vi "Main.vi"(8 "error in (no error)":errorcluster, 11 "Module_Refs":T2={"ModuleName"=enum."Controller", "Queue"=refnum, "user event"=refnum, "VI Refnum"=refnum, "ShowFP"=FALSE, "StatesTracking Enabled"=FALSE}) -> (0 "error out":errorcluster)   [LabVIEW 2021, in "Sound Manager.lvlib"]
uses:
  Sound Manager.lvlib
  Architecture/Typedefs/Module References.ctl
  Architecture/Typedefs/Enum_Module_Name.ctl
  Architecture/Typedefs/Message.ctl
  Typedefs/Sound Effects.ctl
  Typedefs/States.ctl
  Typedefs/Sound Data.ctl
  <vilib>/sound2/lvsound2.llb/Sound Output Task ID.ctl
  Typedefs/Config.ctl
  <vilib>/event_ctls.llb/usereventprio.ctl
  Architecture/Modules/Configuration/Typedefs/App Cfg DVR.ctl
  Architecture/Typedefs/Application Configuration.ctl
  Architecture/Modules/Module Template/Typedefs/Config.ctl
  Architecture/Modules/Core UI/Typedefs/Config.ctl
  Utilities/Globales Snake.vi
  SubVIs/Read Sound ConfigurationI.vi
  Architecture/Architecture.lvlib
  Architecture/Modules/Configuration/Configuration.lvlib
  Architecture/Modules/Module Template/Module Template.lvlib
  Architecture/Modules/Core UI/Board Game.lvlib
panel:
  out "BackGround Track":string
  in  "Next":bool
  in  "Multicolumn Listbox":i32(listbox)
  in  "Stop Sound Effect":bool
  in  "Play Sound Effect":bool
  in  "Sound Effect":T1
  in  "Background music":bool
  in  "Load Config":bool
  out "Message":string
  in  "Stop App":bool
  in  "Stop Module":bool
  # "#Architecture\n\nPlace inside this box all visible data."
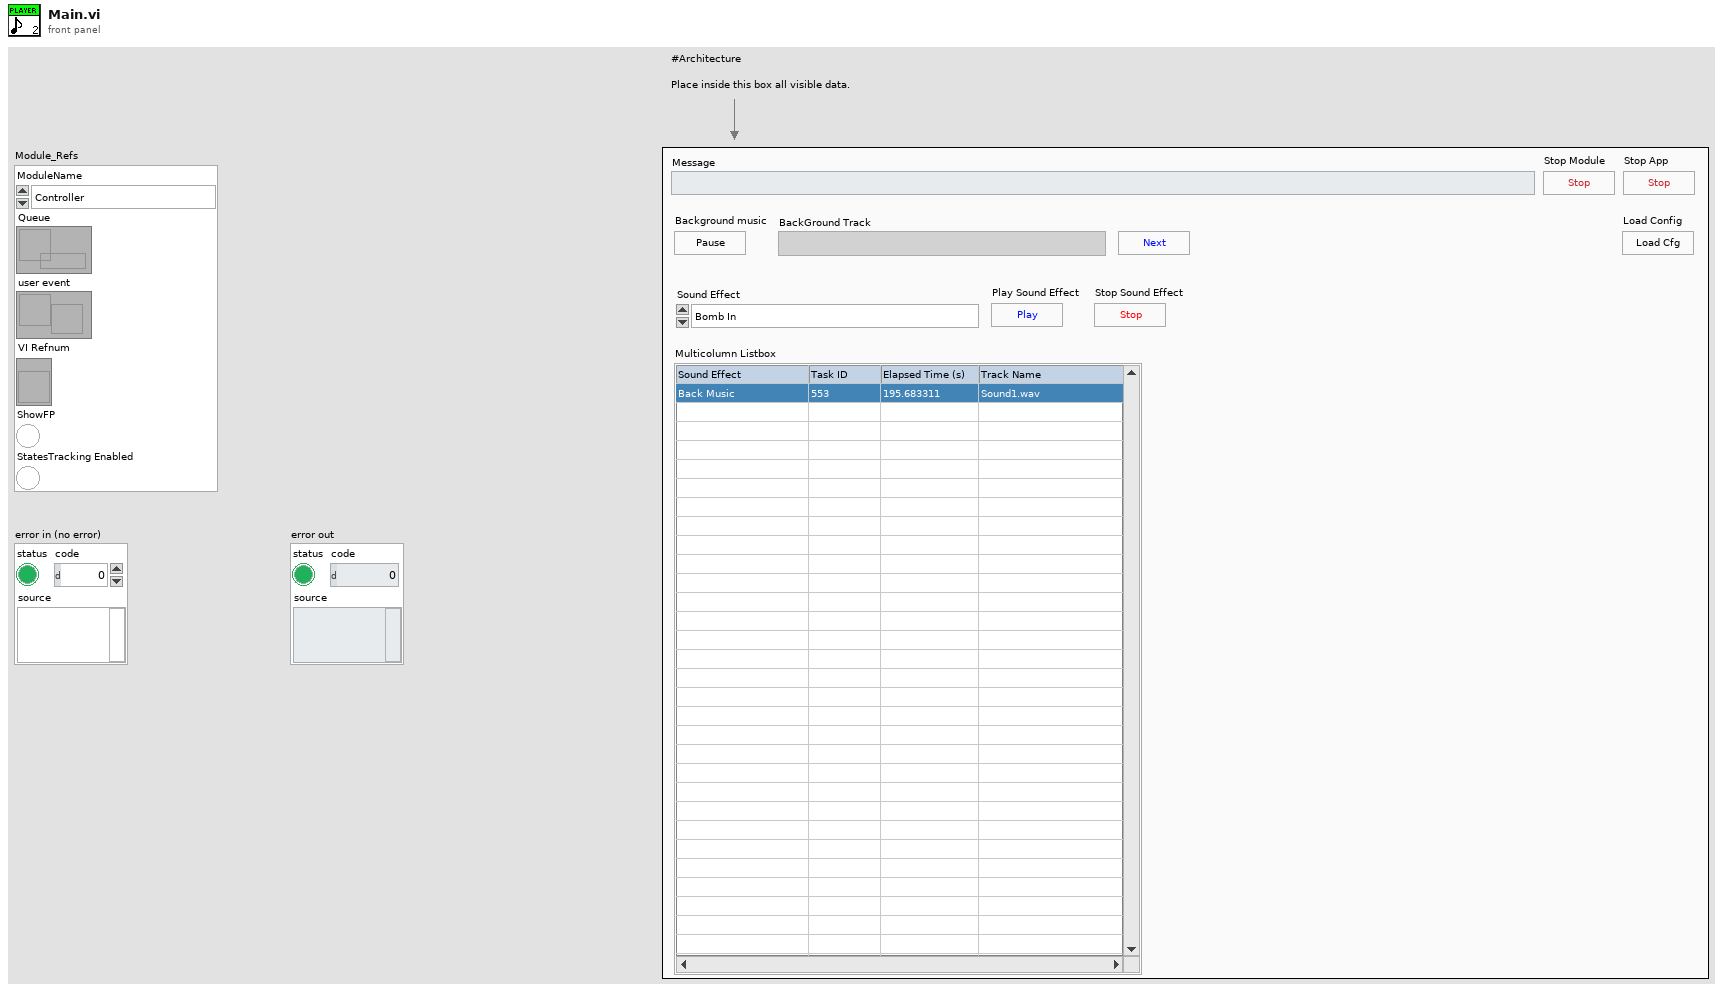
[diagram p1: front panel]
types:
  T1 = typedef "Sound Manager.lvlib/Sound Effects.ctl" = enum16{"Bomb In", "Bomb Out", "Bomb Touched", "Game Over", "Victory", "Eat", "10 Fruits", "Eat2", "Eat3", "Eat4", "MaxShield", "Shield", "10p", "Grape In", "Grape Out", "20p", "30p", "40p", "50p", "60p", "70p", "80p", "90p", "100p", "All shields cracked", "Mouse In", "Mouse Out", "Mouse Eaten", "Grape Eaten", "States Recover", "Broken Shield", "Bonus", "Happy Time", "explode", "Game over musica", "Back Music", "Shield Catch", "Evil lough", "Cricket In", "Cricket eaten", "Lets Go", "Jump1", "Jump2", "Jump3", "Unstoppable", "Troll Music", "winner", "menu"}
  T2 = typedef "Architecture.lvlib/Module References.ctl" = cluster{"ModuleName":T3, "Queue":refnum<queue>, "user event":refnum<user-event>, "VI Refnum":refnum<vi>, "ShowFP":bool, "StatesTracking Enabled":bool}
  T3 = typedef "Configuration.lvlib/Enum_Module_Name.ctl" = enum16{"Configuration", "Error_Handler", "Log", "Database", "Controller", "UI Module", "Sound Manager"}
  T4 = typedef "Sound Manager.lvlib/States.ctl" = cluster{"Module_Refs":T2, "Response Data":variant, "Music Paused":bool, "Tasks":T5[], "Config":T7, "Background Track":string}
  T5 = typedef "Sound Manager.lvlib/Sound Data.ctl" = cluster{"Sound Effect":T1, "Task ID":T6, "Init":timestamp, "Track Name":string}
  T6 = typedef "Sound Output Task ID.ctl" = u32
  T7 = typedef "Sound Manager.lvlib/Config.ctl" = cluster{"Sound Library Path":path, "dyn sounds path":path}
  T8 = enum32{"Invalid", "Standard", "Closed", "Hidden", "Minimized", "Maximized"}
  T9 = typedef "Error_Manager.lvlib/LogRotate.lvclass/LogData.ctl" = cluster{"error in":errorcluster, "replacements":string[], "Time Stamp":timestamp}
  T10 = typedef "Configuration.lvlib/App Cfg DVR.ctl" = refnum<data-value>
  T11 = typedef "usereventprio.ctl" = enum32{"high priority", "normal priority"}
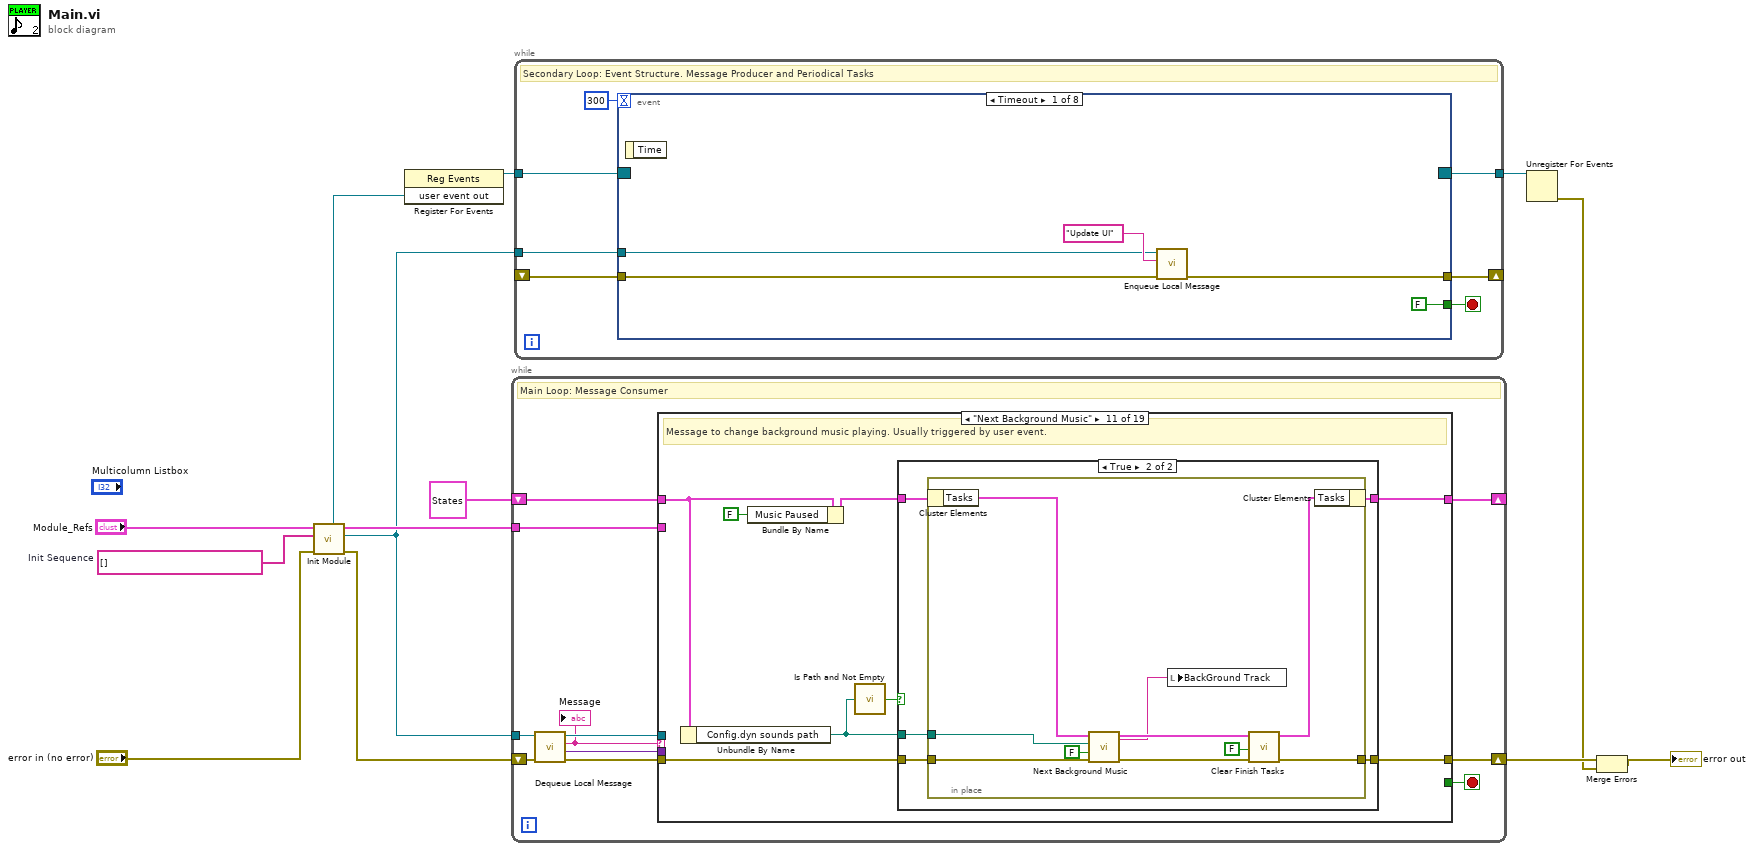
[diagram p0: block diagram]
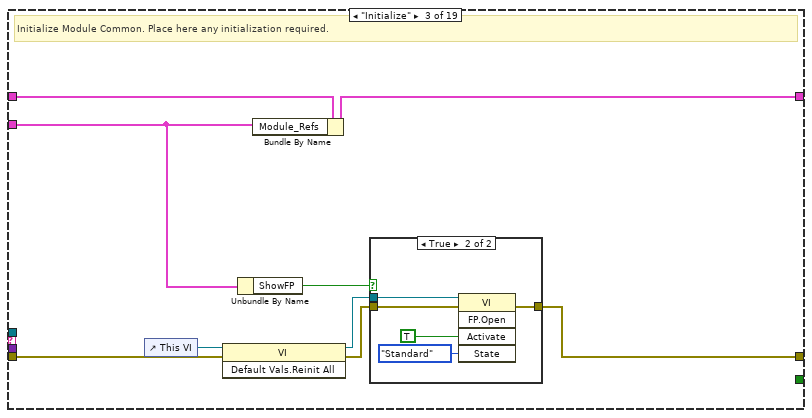
[diagram p4: hidden frame]
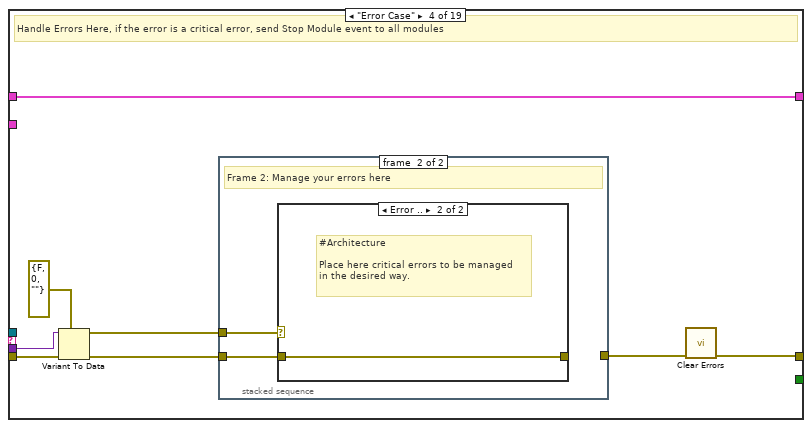
[diagram p6: hidden frame]
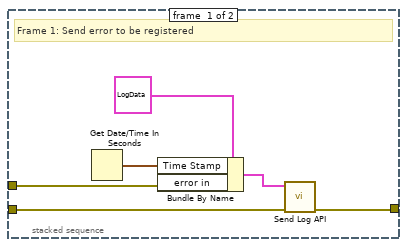
[diagram p7: hidden frame]
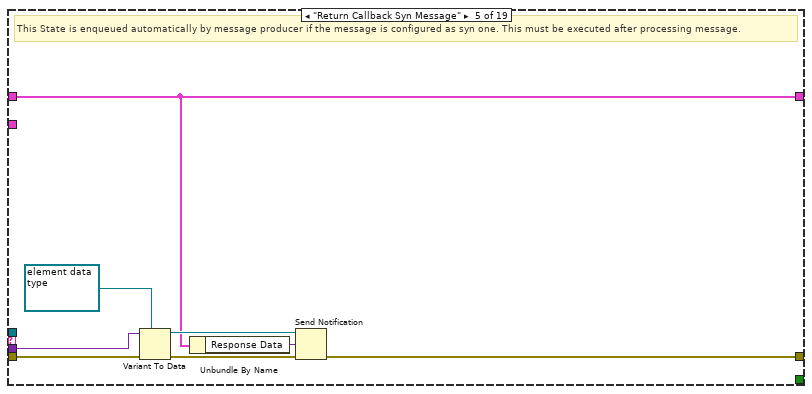
[diagram p9: hidden frame]
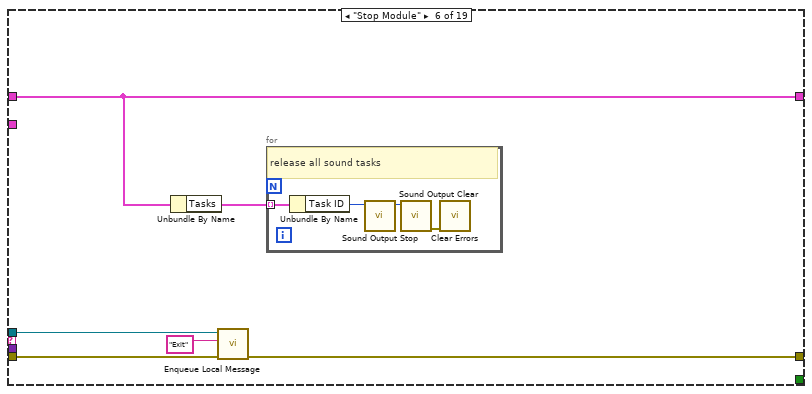
[diagram p10: hidden frame]
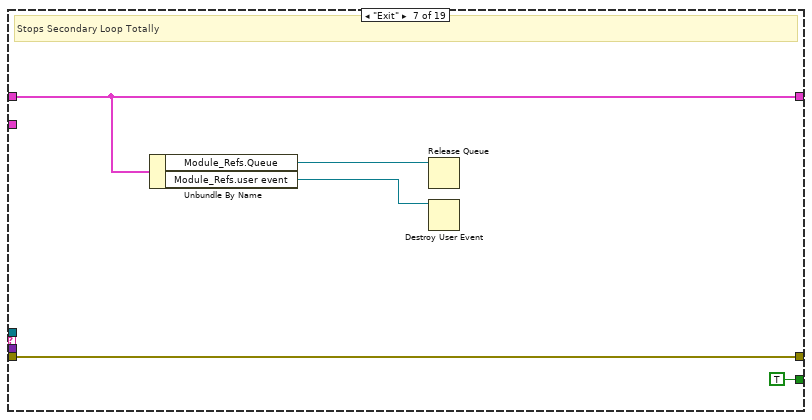
[diagram p11: hidden frame]
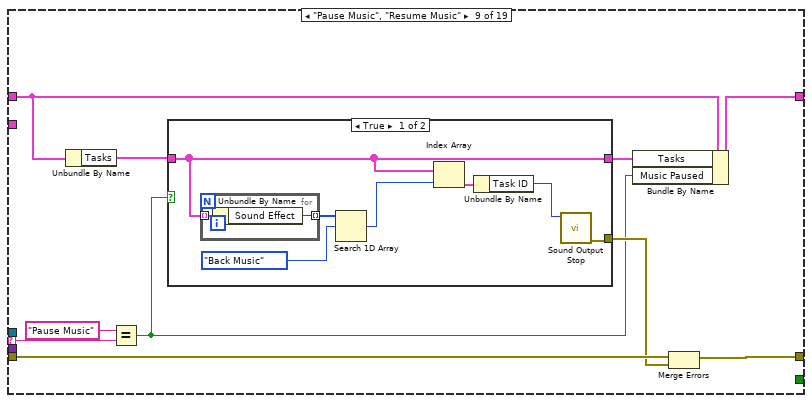
[diagram p13: hidden frame]
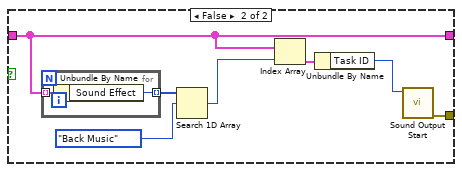
[diagram p14: hidden frame]
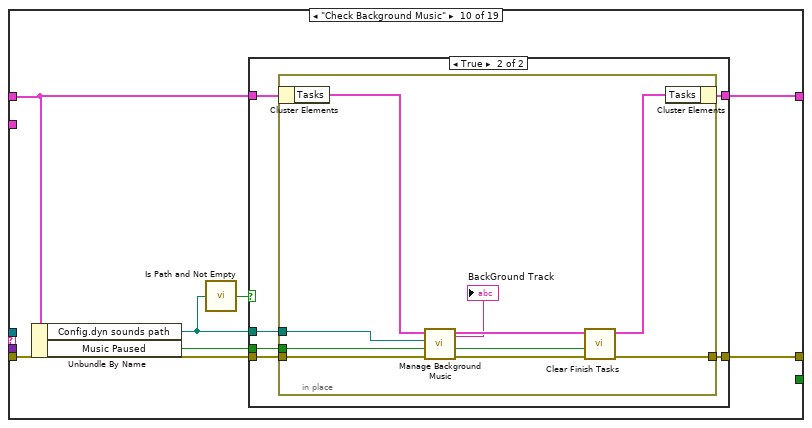
[diagram p15: hidden frame]
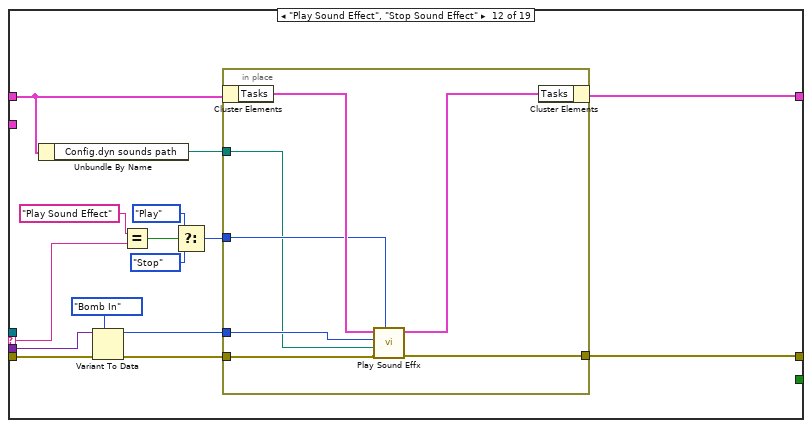
[diagram p18: hidden frame]
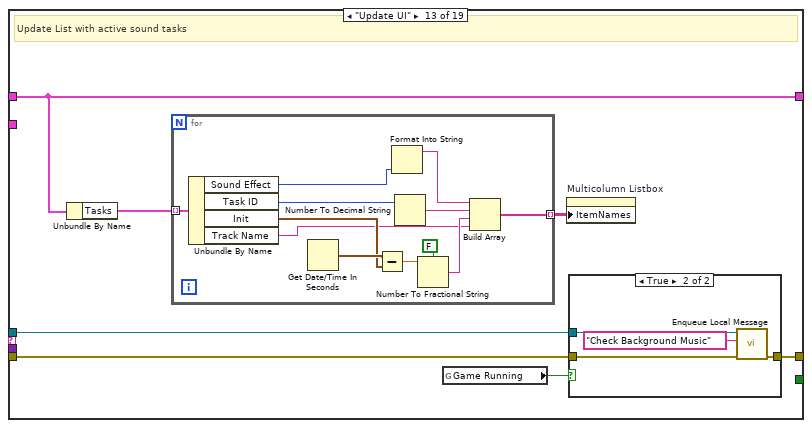
[diagram p19: hidden frame]
diagram:
  w11 = string[] []  # Init Sequence
  n1 = call "Init Module.vi"("error in (no error)"="error in (no error)", "Init Sequence"=w11, "Module Refs"="Module_Refs") -> ("error out"=w13:errorcluster, "queue out"=w2:refnum<queue>, "Module Refs Out"=w4:T2, "user event out"=w3:refnum<user-event>)  [unwired: 5 in]
  n2 = register-events(w3) -> (reference out=w10:refnum<event-registration>)  [unwired: 2 in, 1 out]
  n3 = while {
    shift-right: [w23] -> _
    shift-left: T4 {"Module_Refs"={"ModuleName"=enum."Controller", "Queue"=refnum, "user event"=refnum, "VI Refnum"=refnum, "ShowFP"=FALSE, "StatesTracking Enabled"=FALSE}, "Response Data"=variant, "Music Paused"=FALSE, "Tasks"=[], "Config"={"Sound Library Path"=path "", "dyn sounds path"=path ""}, "Background Track"=""} ("SM Data") -> [w24]
    shift-right: [w22] -> w8
    shift-left: w13 -> [w20]
    tunnel: w2 -> [w21]
    tunnel: w4 -> [w14]
    stop <- w15 stop-if-true
    # "Main Loop: Message Consumer"
    n4 = call "Dequeue Local Message.vi"("error in"=w20, "Msg queue in"=w21) -> ("error out"=w19:errorcluster, "Data"=w16:variant, "Message"=w17:string, "queue out"=w18:refnum<queue>)  [unwired: 6 in]
    "Message" <- w17
    n5 = case shown="\"Next Background Music\"" w17 {
      selector: w17 -> [_ _ _ _ _ _ _ _ w94 _ _ w171 _ _ w212 _ _ _ w256]
      tunnel: w24 -> [w26 w28 w37 w51 w63 w71 w82 w86 w92 w118 w144 w175 w192 w211 w219 w224 w229 w247 w261]
      tunnel: [w26 w28 w35 w51 w63 w71 w82 w86 w95 w117 w143 w173 w192 w211 w219 w224 w225 w247 w261] -> w23
      tunnel: w19 -> [w25 w27 w36 w50 w69 w75 w84 w85 w96 w120 w146 w178 w188 w210 w216 w223 w228 w246 w260]
      tunnel: [w25 w27 w31 w44 w68 w74 w84 w85 w89 w119 w145 w172 w187 w210 w213 w222 w226 w246 w250] -> w22
      tunnel: w18 -> [_ _ _ _ _ w73 _ _ _ _ _ _ w189 _ w214 w221 _ _ w257]
      tunnel: w16 -> [_ _ _ w49 w66 _ _ _ _ _ _ w177 _ _ w215 _ w227 _ w258]
      tunnel: [_ _ _ _ _ _ TRUE _ _ _ _ _ _ _ _ _ _ _ _] -> w15
      tunnel: w14 -> [_ _ w34 _ _ _ _ _ _ _ _ _ _ _ _ _ _ _ _]
      frame "--------State Machine Arquitechture Operations--------" {
      }
      frame "Idle", Default {
        # "Use this state to make iterations if required."
      }
      frame "Initialize" {
        # "Initialize Module Common. Place here any initialization required."
        n6 = control-ref of="This VI"() -> (w29:refnum<vi>)
        n7 = invoke class="VI" method="Default Vals.Reinit All"(reference=w29, error in=w36) -> (reference out=w32:refnum<vi>, error out=w33:errorcluster)  [unwired: 1 in, 1 out]
        n8 = Unbundle By Name(w34) -> ("ShowFP"=w30:bool)
        n9 = Bundle By Name(cluster=w37, "Module_Refs"=w34) -> (w35:T4)
        n10 = case shown="True" w30 {
          tunnel: w33 -> [w38 w43]
          tunnel: [w38 w42] -> w31
          tunnel: w32 -> [_ w41]
          frame False {
          }
          frame True {
            n11 = invoke class="VI" method="FP.Open"(reference=w41, error in=w43, "Activate"=TRUE ("Activate?"), "State"=T8."Standard") -> (error out=w42:errorcluster)  [unwired: 1 in, 4 out]
          }
        }
      }
      frame "Error Case" {
        # "Handle Errors Here, if the error is a critical error, send Stop Module event to all modules"
        n12 = Variant To Data(error in=w50, type=errorcluster {"status"=FALSE, "code"=0, "source"=""} ("error constant"), Variant=w49) -> (data=w45:errorcluster, error out=w47:errorcluster)
        n13 = stacked-sequence {
          tunnel: w47 -> [w57 w59]
          tunnel: [w56 _] -> w46
          tunnel: w45 -> [w54 w58]
          frame #0 {
            # "Frame 1: Send error to be registered"
            n14 = Get Date/Time In Seconds() -> (seconds since 1Jan1904=w53:timestamp)
            n15 = Bundle By Name(cluster=T9 {"error in"={"status"=FALSE, "code"=0, "source"=""}, "replacements"=[], "Time Stamp"=timestamp(0 s since 1904-01-01)} ("Data"), "Time Stamp"=w53, "error in"=w54) -> (w52:T9)
            n16 = call "Send Log API.vi"("error in (no error)"=w57, "Data"=w52) -> ("error out"=w56:errorcluster)  [unwired: 9 in]
          }
          frame #1 {
            # "Frame 2: Manage your errors here"
            n17 = case shown="Error .." w58 {
              tunnel: [w60 w61] -> _
              tunnel: w59 -> [w60 w61]
              frame No Error {
              }
              frame Error {
                # "#Architecture \n\nPlace here critical errors to be managed \nin the desired way."
              }
            }
          }
        }
        n18 = call <vilib>:"Clear Errors.vi"("error in (no error)"=w46) -> ("error out"=w44:errorcluster)  [unwired: 5 in, 1 out]
      }
      frame "Return Callback Syn Message" {
        # "This State is enqueued automatically by message producer if the message is configured as syn one. This must be executed after processing message."
        n19 = Variant To Data(error in=w69, type=refnum<notifier> refnum ("notifier out"), Variant=w66) -> (data=w64:refnum<notifier>, error out=w67:errorcluster)
        n20 = Unbundle By Name(w63) -> ("Response Data"=w62:variant)
        n21 = Send Notification(notification=w62, notifier=w64, error in (no error)=w67) -> (error out=w68:errorcluster)  [unwired: 1 out]
      }
      frame "Stop Module" {
        n22 = Unbundle By Name(w71) -> ("Tasks"=w70:T5[])
        n23 = call "Enqueue Local Message.vi"("error in"=w75, "Message"="Exit", "Msg queue in"=w73) -> ("error out"=w74:errorcluster)  [unwired: 7 in, 1 out]
        n24 = for {
          tunnel: w70 -> [w77] mode=indexing
          # "release all sound tasks"
          n25 = Unbundle By Name(w77) -> ("Task ID"=w76:T6)
          n26 = call <vilib>:"Sound Output Stop.vi"("task ID"=w76) -> ("task ID out"=w78:T6)  [unwired: 9 in, 1 out]
          n27 = call <vilib>:"Sound Output Clear.vi"("task ID"=w78) -> ("error out"=w79:errorcluster)  [unwired: 10 in]
          n28 = call <vilib>:"Clear Errors.vi"("error in (no error)"=w79) -> ()  [unwired: 5 in, 2 out]
        }
      }
      frame "Exit" {
        # "Stops Secondary Loop Totally"
        n29 = Unbundle By Name(w82) -> ("Module_Refs.Queue"=w81:refnum<queue>, "Module_Refs.user event"=w80:refnum<user-event>)
        n30 = Release Queue(queue=w81) -> ()  [unwired: 2 in, 3 out]
        n31 = Destroy User Event(user event=w80) -> ()  [unwired: 1 in, 1 out]
      }
      frame "--------------State Machine Custom States-------------" {
      }
      frame "Pause Music", "Resume Music" {
        n32 = Unbundle By Name(w92) -> ("Tasks"=w91:T5[])
        n33 = Equal?(x="Pause Music", y=w94) -> (x = y?=w87:bool)
        n34 = case shown="True" w87 {
          tunnel: w91 -> [w99 w109]
          tunnel: [w99 w109] -> w90
          tunnel: [w97 w107] -> w88
          frame True {
            n35 = for {
              tunnel: w99 -> [w105] mode=indexing
              tunnel: [w104] -> w101 mode=indexing
              n36 = Unbundle By Name(w105) -> ("Sound Effect"=w104:T1)
            }
            n37 = Search 1D Array(1D array=w101, element=Sound_Effects."Back Music") -> (index of element=w100:i32)  [unwired: 1 in]
            n38 = Index Array(array=w99, index=w100) -> (element=w103:T5)
            n39 = Unbundle By Name(w103) -> ("Task ID"=w98:T6)
            n40 = call <vilib>:"Sound Output Stop.vi"("task ID"=w98) -> ("error out"=w97:errorcluster)  [unwired: 9 in, 1 out]
          }
          frame False {
            n41 = for {
              tunnel: w109 -> [w114] mode=indexing
              tunnel: [w113] -> w111 mode=indexing
              n42 = Unbundle By Name(w114) -> ("Sound Effect"=w113:T1)
            }
            n43 = Search 1D Array(1D array=w111, element=Sound_Effects."Back Music" ("Sound Effect")) -> (index of element=w110:i32)  [unwired: 1 in]
            n44 = Index Array(array=w109, index=w110) -> (element=w112:T5)
            n45 = Unbundle By Name(w112) -> ("Task ID"=w108:T6)
            n46 = call <vilib>:"Sound Output Start.vi"("task ID"=w108) -> ("error out"=w107:errorcluster)  [unwired: 9 in, 1 out]
          }
        }
        n47 = Bundle By Name(cluster=w92, "Tasks"=w90, "Music Paused"=w87) -> (w95:T4)
        n48 = Merge Errors(w96, w88) -> (w89:errorcluster)
      }
      frame "Check Background Music" {
        n49 = Unbundle By Name(w118) -> ("Config.dyn sounds path"=w116:path, "Music Paused"=w121:bool)
        n50 = call <vilib>:"Is Path and Not Empty.vi"("path"=w116) -> ("Is Path and Not Empty?"=w115:bool)  [unwired: 4 in]
        n51 = case shown="True" w115 {
          tunnel: w121 -> [_ w129]
          tunnel: w120 -> [w122 w128]
          tunnel: [w122 w124] -> w119
          tunnel: w118 -> [w123 w127]
          tunnel: [w123 w126] -> w117
          tunnel: w116 -> [_ w125]
          frame False {
          }
          frame True {
            n52 = in-place {
              in-place-border: w129 -> [w131]
              in-place-border: w128 -> [w136]
              in-place-border: w125 -> [w135]
              in-place-border: [w138] -> w124
              n53 = in-place-cluster #1(w127) -> ("Tasks"=w134:T5[])
              n54 = call "Manage Background Music.vi"("error in (no error)"=w136, "Music Paused"=w131, "Dyn Sounds Path"=w135, "Sounds"=w134) -> ("error out"=w137:errorcluster, "Sounds Out"=w133:T5[], "BackGround Track"=→"BackGround Track":string)  [unwired: 5 in]
              n55 = call "Clear Finish Tasks.vi"("error out"=w137, "Music Paused"=w131, "Sounds In"=w133) -> ("error out"=w138:errorcluster, "Sounds Out"=w132:T5[])  [unwired: 7 in]
              n56 = in-place-cluster #1("Tasks"=w132) -> (w126:T4)
            }
          }
        }
      }
      frame "Next Background Music" {
        # "Message to change background music playing. Usually triggered by user event."
        n57 = Unbundle By Name(w144) -> ("Config.dyn sounds path"=w142:path)
        n58 = Bundle By Name(cluster=w144, "Music Paused"=FALSE) -> (w140:T4)
        n59 = call <vilib>:"Is Path and Not Empty.vi"("path"=w142) -> ("Is Path and Not Empty?"=w141:bool)  [unwired: 4 in]
        n60 = case shown="True" w141 {
          tunnel: w146 -> [w147 w153]
          tunnel: [w147 w152] -> w145
          tunnel: w140 -> [w148 w151]
          tunnel: [w148 w150] -> w143
          tunnel: w142 -> [_ w149]
          frame False {
          }
          frame True {
            n61 = in-place {
              in-place-border: w153 -> [w156]
              in-place-border: [w161] -> w152
              in-place-border: w149 -> [w157]
              n62 = in-place-cluster #2(w151) -> ("Tasks"=w159:T5[])
              n63 = call "Next Background Music.vi"("error in (no error)"=w156, "Music Paused"=FALSE, "Dyn Sounds Path"=w157, "Sounds"=w159) -> ("error out"=w163:errorcluster, "Sounds Out"=w162:T5[], "BackGround Track"=w158:string)  [unwired: 5 in]
              n64 = local write "BackGround Track"(w158) -> ()
              n65 = call "Clear Finish Tasks.vi"("error out"=w163, "Music Paused"=FALSE, "Sounds In"=w162) -> ("error out"=w161:errorcluster, "Sounds Out"=w160:T5[])  [unwired: 7 in]
              n66 = in-place-cluster #2("Tasks"=w160) -> (w150:T4)
            }
          }
        }
      }
      frame "Play Sound Effect", "Stop Sound Effect" {
        n67 = Unbundle By Name(w175) -> ("Config.dyn sounds path"=w174:path)
        n68 = Variant To Data(error in=w178, type=Sound_Effects."Bomb In" ("Sound Effect Off"), Variant=w177) -> (data=w164:T1, error out=w176:errorcluster)
        n69 = Equal?(x="Play Sound Effect", y=w171) -> (x = y?=w169:bool)
        n70 = Select(t=enum16{"Play", "Stop"}."Play" ("event"), s=w169, f=enum16{"Play", "Stop"}."Stop" ("event")) -> (s? t:f=w166:enum16{"Play", "Stop"})
        n71 = in-place {
          in-place-border: w176 -> [w185]
          in-place-border: w174 -> [w180]
          in-place-border: [w179] -> w172
          in-place-border: w166 -> [w182]
          in-place-border: w164 -> [w181]
          n72 = in-place-cluster #3(w175) -> ("Tasks"=w184:T5[])
          n73 = call "Play Sound Effx.vi"("event"=w182, "error in (no error)"=w185, "path"=w180, "Sound Effect Off"=w181, "Sounds In"=w184) -> ("error out"=w179:errorcluster, "Sounds Out"=w183:T5[])  [unwired: 5 in]
          n74 = in-place-cluster #3("Tasks"=w183) -> (w173:T4)
        }
      }
      frame "Update UI" {
        # "Update List with active sound tasks"
        n75 = Unbundle By Name(w192) -> ("Tasks"=w191:T5[])
        n76 = for {
          tunnel: w191 -> [w209] mode=indexing
          tunnel: [w199] -> w190 mode=indexing
          n77 = Unbundle By Name(w209) -> ("Sound Effect"=w208:T1, "Task ID"=w206:T6, "Init"=w203:timestamp, "Track Name"=w198:string)
          n78 = Get Date/Time In Seconds() -> (seconds since 1Jan1904=w204:timestamp)
          n79 = Subtract(x=w204, y=w203) -> (x-y=w202:dbl)
          n80 = Format Into String(w208) -> (resulting string=w207:string)  [unwired: 3 in, 1 out]
          n81 = Number To Decimal String(number=w206) -> (decimal integer string=w205:string)  [unwired: 1 in]
          n82 = Number To Fractional String(use system decimal point (T)=FALSE, number=w202) -> (F-format string=w200:string)  [unwired: 2 in]
          n83 = Build Array(w207, w205, w200, w198) -> (w199:string[])
        }
        n84 = global read "Globales Snake.vi" "Game Running"() -> (w186:bool)
        n85 = property on="Multicolumn Listbox" class="MCListbox (strict)"("ItemNames"=w190) -> ()  [unwired: 2 in, 2 out]
        n86 = case shown="True" w186 {
          tunnel: w189 -> [_ w196]
          tunnel: w188 -> [w193 w195]
          tunnel: [w193 w194] -> w187
          frame False {
          }
          frame True {
            n87 = call "Enqueue Local Message.vi"("error in"=w195, "Message"="Check Background Music", "Msg queue in"=w196) -> ("error out"=w194:errorcluster)  [unwired: 7 in, 1 out]
          }
        }
      }
      frame "--------------Dynamic Events Messages----------------" {
      }
      frame "Message: Check Background Music", "Message: MyMessage", "Message: Next Background Music", "Message: Pause Music", "Message: Play Sound Effect", "Message: Resume Music", "Message: Stop Sound Effect" {
        n88 = Match Pattern(string=w212, regular expression="Message: ") -> (after substring=w217:string)  [unwired: 1 in, 3 out]
        n89 = call "Enqueue Local Message.vi"("error in"=w216, "Data"=w215, "Message"=w217, "Msg queue in"=w214) -> ("error out"=w213:errorcluster)  [unwired: 6 in, 1 out]
      }
      frame "Message: Stop Module" {
        n90 = call "Enqueue Local Message.vi"("error in"=w223, "Message"="Stop Module", "Msg queue in"=w221) -> ("error out"=w222:errorcluster)  [unwired: 7 in, 1 out]
      }
      frame "Message: Load Config" {
        # "Message used to receive configuration from a configuration module. Decode dedicated typedef and save it into SM Data"
        n91 = disable-structure shown="Simulation==False, Default" {
          disable-tunnel: w229 -> [w238 w244]
          disable-tunnel: w228 -> [w237 w245]
          disable-tunnel: w227 -> [w236 _]
          disable-tunnel: [w230 _] -> w226
          disable-tunnel: [_ w245] -> _
          disable-tunnel: [w234 w243] -> w225
          frame condition #0 (active) {
            n92 = Variant To Data(error in=w237, type=T10 refnum ("App Cfg DVR"), Variant=w236) -> (data=w233:T10, error out=w232:errorcluster)
            n93 = call-poly "POLY Read Configuration API.vi"("error constant"=w232, "App Cfg DVR"=w233) -> ("error out"=w230:errorcluster, "Sound Manager Config"=w231:T7)  [unwired: 8 in]
            n94 = Bundle By Name(cluster=w238, "Config"=w231) -> (w234:T4)
          }
          frame condition #1 {
            n95 = call <vilib>:"Application Directory.vi"() -> ("Application Directory"=w242:path)
            n96 = Build Path(base path=w242, name or relative path=path "Resources/sounds/%s.wav") -> (appended path=w240:path)
            n97 = Strip Path(path=w240) -> (stripped path=w239:path)  [unwired: 1 out]
            n98 = Bundle By Name(cluster=w244, "Config.Sound Library Path"=w239, "Config.dyn sounds path"=w240) -> (w243:T4)
          }
        }
      }
      frame "------------Synchronous Event Messages--------------" {
      }
      frame "SynMessage: MySynMessage" {
        # "Use this case as a handler for Synchronous messages. This state queues a message for the desired"
        n99 = call "Extract Synchronous Data.vi"("error in 2"=w260, "Variant"=w258) -> ("error in"=w259:errorcluster, "Data Out"=w253:variant, "notifier out"=w248:refnum<notifier>)  [unwired: 7 in]
        n100 = Match Pattern(string=w256, regular expression="SynMessage: ") -> (after substring=w254:string)  [unwired: 1 in, 3 out]
        n101 = call "Enqueue Local Message.vi"("error in"=w259, "Data"=w253, "Message"=w254, "Msg queue in"=w257) -> ("error out"=w252:errorcluster, "queue out"=w251:refnum<queue>)  [unwired: 6 in]
        n102 = call "Enqueue Local Message.vi"("error in"=w252, "Data"=w248, "Message"="Return Callback Syn Message", "Msg queue in"=w251) -> ("error out"=w250:errorcluster)  [unwired: 6 in, 1 out]
      }
    }
  }
  n103 = while {
    tunnel: w10 -> [w268]
    tunnel: w2 -> [w265]
    tunnel: [w264] -> w9
    shift-right: [w262] -> _
    shift-left: _ -> [w263]
    stop <- w266 stop-if-true
    # "Secondary Loop: Event Structure. Message Producer and Periodical Tasks"
    n104 = event shown="[0] Timeout" {
      selector: w268 -> [_ _ _ _ _ _ _ _]
      dyn-events: [_ _ _ _ _ _ _ _] -> w264
      timeout: 300 -> [_ _ _ _ _ _ _ _]
      tunnel: [FALSE w280 TRUE _ _ _ _ _] -> w266
      tunnel: w265 -> [w269 w285 w287 _ _ _ _ _]
      tunnel: w263 -> [w270 w284 w290 w292 w301 w309 w317 w324]
      tunnel: [w271 w283 w288 w291 w300 w308 w318 w323] -> w262
      event Timeout {
        n105 = event-data() -> ()  [unwired: 1 in, 1 out]
        n106 = call "Enqueue Local Message.vi"("error in"=w270, "Message"="Update UI", "Msg queue in"=w269) -> ("error out"=w271:errorcluster)  [unwired: 7 in, 1 out]
      }
      event User Event {
        # "Send message to local queue. \n(Message Consumer)"
        # "Processes an external event and enqueues a message to the local queue. It can be synchronous (with response) or NOT."
        n107 = event-data() -> ("syn"=w277:bool, "Message"=w279:string, "Data"=w282:variant)  [unwired: 1 in]
        n108 = Select(t="SynMessage: " ("string"), s=w277, f="Message: " ("string")) -> (s? t:f=w274:string)
        n109 = Concatenate Strings(w274, w279) -> (w281:string)
        n110 = call "Enqueue Local Message.vi"("error in"=w284, "Data"=w282, "Message"=w281, "Msg queue in"=w285) -> ("error out"=w283:errorcluster)  [unwired: 6 in, 1 out]
        n111 = Equal?(x=w279, y="Stop Module") -> (x = y?=w280:bool)
      }
      event "Stop Module": Value Change {
        n112 = event-data() -> ()  [unwired: 1 in, 1 out]
        n113 = call "Enqueue Local Message.vi"("error in"=w290, "Message"="Stop Module", "Msg queue in"=w287) -> ("error out"=w288:errorcluster)  [unwired: 7 in, 1 out]
      }
      event "Stop App": Value Change {
        w294 = TRUE  # All Modules
        # "Send Stop To All Modules"
        n114 = event-data() -> ()  [unwired: 1 in, 1 out]
        n115 = call "Send Message Modules.vi"("All Modules"=w294, "Error In"=w292, "Message"="Stop Module") -> ("error in (no error)"=w291:errorcluster)  [unwired: 8 in]
      }
      event "Load Config": Value Change {
        n116 = event-data() -> ()  [unwired: 1 in, 1 out]
        n117 = To Variant(anything=T10 refnum ("App Cfg DVR")) -> (Variant=w298:variant)
        n118 = call "Send Message Module.vi"("priority (normal)"=usereventprio."high priority", "Error In"=w301, "Data"=w298, "Message"="Load Config", "Target ModuleName In"=Enum_Module_Name."Sound Manager" ("ModuleName")) -> ("error in (no error)"=w300:errorcluster)  [unwired: 6 in]
      }
      event "Background music": Value Change {
        n119 = event-data() -> ("NewVal"=w306:bool)  [unwired: 1 in]
        n120 = Select(t="Pause Music", s=w306, f="Resume Music") -> (s? t:f=w303:string)
        n121 = call "Send Message Module.vi"("priority (normal)"=usereventprio."normal priority", "Error In"=w309, "Message"=w303, "Target ModuleName In"=Enum_Module_Name."Sound Manager" ("ModuleName")) -> ("error in (no error)"=w308:errorcluster)  [unwired: 7 in]
      }
      event "Play Sound Effect", "Stop Sound Effect": Value Change {
        n122 = event-data() -> ("CtlRef"=w319:refnum<vi>)  [unwired: 1 in]
        n123 = property class="Bool"(reference=w319) -> ("Label.Text"=w315:string)  [unwired: 1 in, 2 out]
        n124 = Equal?(x=w315, y="Stop") -> (x = y?=w313:bool)
        n125 = Boolean To (0,1)(Boolean=w313) -> (0, 1=w312:i16)
        n126 = Type Cast(type=enum16{"Play", "Stop"}."Play" ("Function"), x=w312) -> (*(type *) &x=w310:enum16{"Play", "Stop"})
        n127 = call "Play Stop Sound Effx.vi"("Sound Effect"="Sound Effect", "Error In"=w317, "Function"=w310) -> ("error in (no error)"=w318:errorcluster)  [unwired: 8 in]
      }
      event "Next": Value Change {
        n128 = event-data() -> ()  [unwired: 1 in, 1 out]
        n129 = call "Send Message Module.vi"("priority (normal)"=usereventprio."high priority", "Error In"=w324, "Message"="Next Background Music", "Target ModuleName In"=Enum_Module_Name."Sound Manager") -> ("error in (no error)"=w323:errorcluster)  [unwired: 7 in]
      }
    }
  }
  n130 = Unregister For Events(event registration refnum=w9) -> (error out=w7:errorcluster)  [unwired: 1 in]
  n131 = Merge Errors(w8, w7) -> (→"error out":errorcluster)
